vi "Lab4_task3.vi"() -> ()   [LabVIEW 2022 SP3]
uses:
  <vilib>/Utility/file.llb/Write Delimited Spreadsheet (DBL).vi
  <vilib>/express/express analysis/Spectral/Block/exnSpectralBlock spectral measurements PSD poly.vi
  <vilib>/express/express analysis/Spectral/Block/exnSpectralBlock spectral measurements PSD DDT.vi
  <vilib>/express/express analysis/Spectral/XNode/ExpressSpectralMeasurementsBlockNode.xnode
  <vilib>/Analysis/NI_AALPro.lvlib
panel:
  out "XY Graph":T1(graph)
  out "PSD":dynamicdata(graph)
  out "Peak-to-peak (V)":dbl
  out "RMS Noise (V)":dbl
  out "Mean Value (V)":dbl
  out "Array":dbl[](array[numeric])
  in  "file path (dialog if empty)":path
  out "Waveform Chart":dynamicdata(graph)
  out "Total execution time (s)":u32
  out "Sampling period (ms)":dbl
  out "Total number of samples":dbl
  in  "Sampling rate (Hz)":dbl
  in  "Total duration (s)":dbl
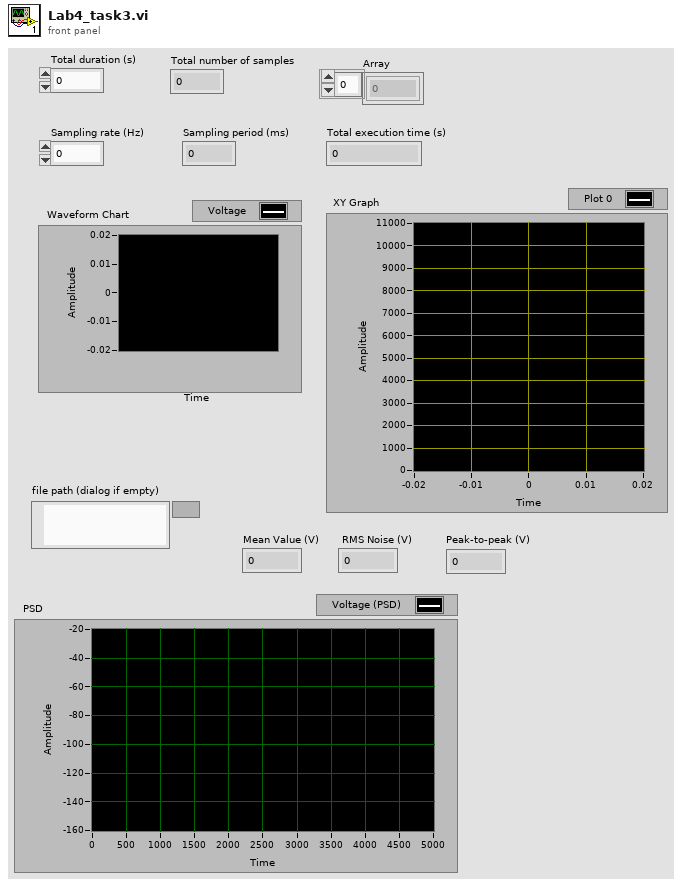
[diagram p1: front panel]
types:
  T1 = cluster{"X Values":dbl[], "Histogram: h(x)":i32[]}
  T2 = cluster{"averaging mode":u16, "weighting mode":u16, "number of averages":u32}
  T3 = cluster{"dB On (F)":bool, "unwrap phase (F)":bool, "convert to degree (F)":bool}
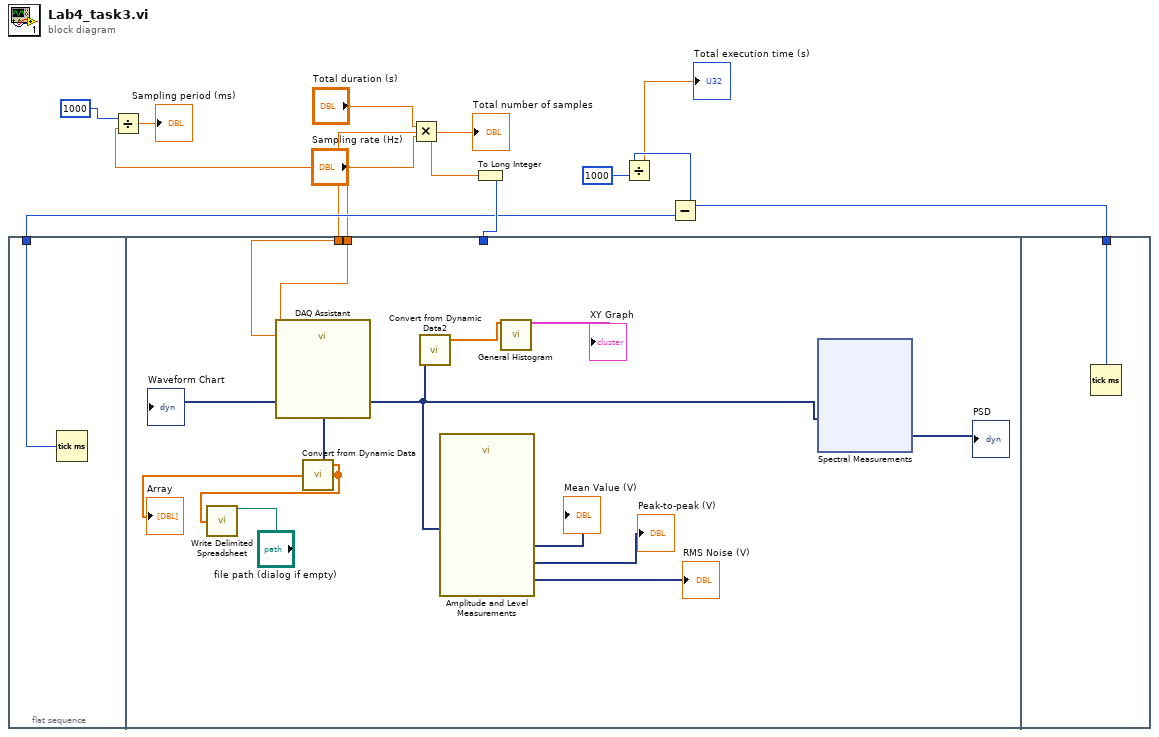
[diagram p0: block diagram]
diagram:
  n1 = flat-sequence {
    tunnel: [w12] -> w4
    tunnel: w9 -> [_]
    tunnel: "Sampling rate (Hz)" -> [w23]
    tunnel: w1 -> [w22]
    tunnel: [w33] -> w5
    frame #0 {
      n2 = Tick Count (ms)() -> (millisecond timer value=w12:u32)
    }
    frame #1 {
      n3 = call "DAQ Assistant"("rate"=w23, "number of samples"=w22) -> ("data"=w17:dynamicdata)  [unwired: 15 in, 2 out]
      "Waveform Chart" <- w17
      n4 = call "Convert from Dynamic Data"("Dynamic Data Type"=w17) -> ("Array"=w21:dbl[])  [unwired: 3 in]
      "Array" <- w21
      n5 = call-poly <vilib>:"Write Delimited Spreadsheet.vi"("file path (dialog if empty)"="file path (dialog if empty)", "1D data"=w21) -> ()  [unwired: 12 in, 2 out]
      n6 = call "Convert from Dynamic Data2"("Dynamic Data Type"=w17) -> ("Array"=w16:dbl[])  [unwired: 3 in]
      n7 = call "Amplitude and Level Measurements"("Signals"=w17) -> ("Mean (DC)"=→"Mean Value (V)":dynamicdata, "RMS"=→"RMS Noise (V)":dynamicdata, "Peak to Peak"=→"Peak-to-peak (V)":dynamicdata)  [unwired: 11 in, 1 out]
      n8 = call <vilib>:"General Histogram.vi"("X"=w16) -> ("Histogram Graph"=→"XY Graph":T1)  [unwired: 10 in, 4 out]
      n9 = xnode "Spectral Measurements"("Signals"=w17) -> ("PSD"=→"PSD":dynamicdata)  [unwired: 1 in, 1 out]
    }
    frame #2 {
      n10 = Tick Count (ms)() -> (millisecond timer value=w33:u32)
    }
  }
  n11 = Divide(x=1000, y="Sampling rate (Hz)") -> (x/y=→"Sampling period (ms)":dbl)
  n12 = Multiply(x="Total duration (s)", y="Sampling rate (Hz)") -> (x*y=w1:dbl)
  "Total number of samples" <- w1
  n13 = To Long Integer(number=w1) -> (32bit integer=w9:i32)
  n14 = Subtract(x=w5, y=w4) -> (x-y=w8:u32)
  n15 = Divide(x=w8, y=u32 1000) -> (x/y=→"Total execution time (s)":dbl)
